vi "Initialize.vi"(8 "error in":errorcluster, 9 "Settings":T1={"Baud Rate"=enum."9600", "Timeout"=2000, "Stop Bits"=10, "Flow Control"=enum."None", "Parity"=0} {"Parity" items=["None", "Odd", "Even", "Mark", "Space"]; "Stop Bits" items=["1.0"=10, "1.5"=15, "2.0"=20]}, 10 "Reset?":bool, 11 "VISA resource name":refnum<visa-resource-name>) -> (0 "error out":errorcluster, 3 "VISA resource name out":refnum<visa-resource-name>)   [LabVIEW 2021, in "Keysight U1282A.lvlib"]
doc: "Este bloque inicializa la interfaz de comunicación serial (VISA) del instrumento U1282A."
uses:
  Keysight U1282A.lvlib
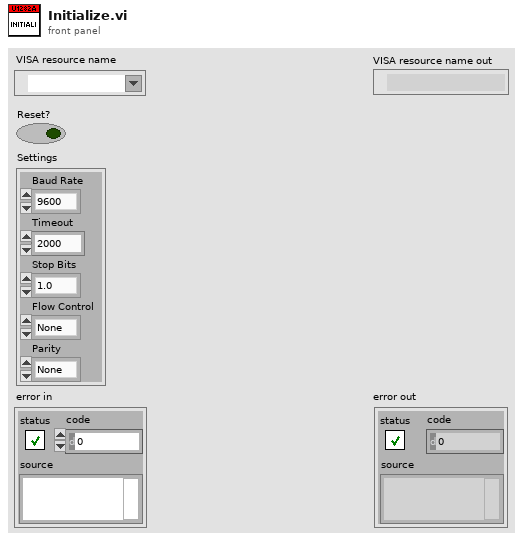
[diagram p1: front panel]
types:
  T1 = cluster{"Baud Rate":enum16{"1200", "2400", "4800", "9600", "19200", "38400", "57600", "115200"}, "Timeout":u32, "Stop Bits":u16, "Flow Control":enum16{"None", "XON / XOFF", "RTS / CTS", "DTR / DSR"}, "Parity":u16}
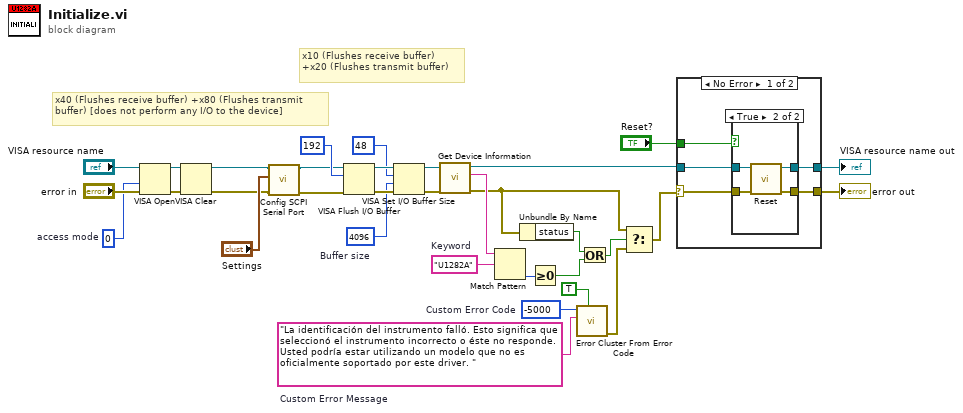
[diagram p0: block diagram]
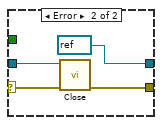
[diagram p3: hidden frame]
diagram:
  w19 = "La identificación del instrumento falló. Esto significa que seleccionó el instrumento incorrecto o éste no responde. Usted podría estar utilizando un modelo que no es oficialmente soportado por este driver. "  # Custom Error Message
  w20 = -5000  # Custom Error Code
  w21 = "U1282A"  # Keyword
  w23 = u32 4096  # Buffer size
  w31 = u32 0  # access mode
  # "x10 (Flushes receive buffer) +x20 (Flushes transmit buffer)"
  # "x40 (Flushes receive buffer) +x80 (Flushes transmit buffer) [does not perform any I/O to the device]"
  n1 = VISA Open(access mode=w31, error in (no error)="error in", VISA resource name="VISA resource name") -> (VISA resource name=w30:refnum<visa-resource-name>, error out=w29:errorcluster)  [unwired: 2 in]
  n2 = VISA Clear(VISA resource name=w30, error in (no error)=w29) -> (VISA resource name out=w10:refnum<visa-resource-name>, error out=w11:errorcluster)
  n3 = call "Config SCPI Serial Port.vi"("error in"=w11, "Settings"="Settings", "VISA Refnum in"=w10) -> ("error out"=w12:errorcluster, "VISA Refnum out"=w13:refnum<visa-resource-name>)  [unwired: 7 in]
  n4 = VISA Flush I/O Buffer(VISA resource name=w13, mask (16)=u16 192, error in (no error)=w12) -> (VISA resource name out=w26:refnum<visa-resource-name>, error out=w25:errorcluster)
  n5 = VISA Set I/O Buffer Size(VISA resource name=w26, mask (16)=u16 48, size (4096)=w23, error in (no error)=w25) -> (VISA resource name out=w5:refnum<visa-resource-name>, error out=w2:errorcluster)
  n6 = call "Get Device Information.vi"("error in"=w2, "VISA resource name in"=w5) -> ("error out"=w3:errorcluster, "Model Number"=w8:string, "VISA resource name out"=w4:refnum<visa-resource-name>)  [unwired: 4 in, 3 out]
  n7 = Match Pattern(string=w8, regular expression=w21) -> (offset past match=w18:i32)  [unwired: 1 in, 3 out]
  n8 = Unbundle By Name(w3) -> ("status"=w17:bool)
  n9 = Greater Or Equal To 0?(x=w18) -> (x >= 0?=w16:bool)
  n10 = call <vilib>:"Error Cluster From Error Code.vi"("show call chain? (False)"=TRUE, "error message (\"\")"=w19, "error code (0)"=w20) -> ("error out"=w6:errorcluster)  [unwired: 6 in]
  n11 = Or(x=w17, y=w16) -> (x .or. y?=w15:bool)
  n12 = Select(t=w3, s=w15, f=w6) -> (s? t:f=w9:errorcluster)
  n13 = case shown="No Error" w9 {
    selector: w9 -> [w35 w47]
    tunnel: [w38 refnum<visa-resource-name> refnum ("VISA resource name out")] -> w28
    tunnel: [w37 w46] -> w27
    tunnel: w4 -> [w36 w45]
    tunnel: "Reset?" -> [w34 _]
    frame No Error {
      n14 = case shown="True" w34 {
        tunnel: [w39 w44] -> w38
        tunnel: [w40 w43] -> w37
        tunnel: w35 -> [w40 w42]
        tunnel: w36 -> [w39 w41]
        frame False {
        }
        frame True {
          n15 = call "Reset.vi"("error in"=w42, "VISA resource name in"=w41) -> ("error out"=w43:errorcluster, "VISA resource name out"=w44:refnum<visa-resource-name>)  [unwired: 7 in, 1 out]
        }
      }
    }
    frame Error {
      n16 = call "Close.vi"("error in"=w47, "VISA resource name"=w45) -> ("error out"=w46:errorcluster)  [unwired: 9 in]
    }
  }
  "VISA resource name out" <- w28
  "error out" <- w27
